vi "Network Steam Create.vi"(8 "error in (no error)":errorcluster, 11 "Model_AMC in":refnum<class "Model_AMC.lvclass">) -> (0 "error out":errorcluster, 3 "Model_AMC out":refnum<class "Model_AMC.lvclass">)   [LabVIEW 2021, in "Model_AMC.lvclass"]
uses:
  Model_AMC.lvclass
  Model_AMC.lvclass/Model_AMC.ctl
  <userlib>/John_Lib/Network_Streams_Connection/NetworkConnection.lvclass
  <userlib>/John_Lib/Network_Streams_Connection/PublicSettings.ctl
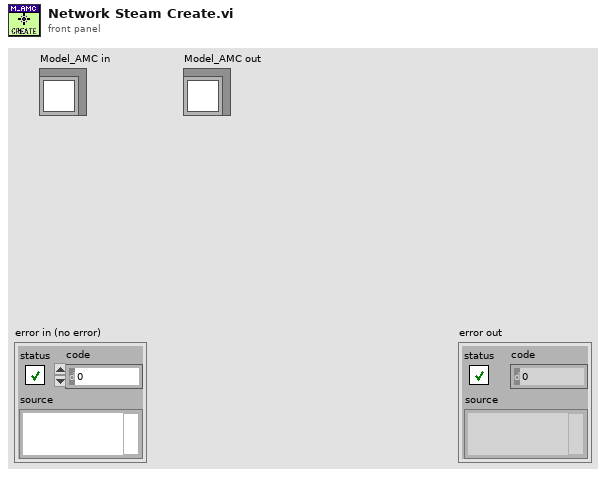
[diagram p1: front panel]
types:
  T1 = typedef "JKI_Network_Streams.lvlib/NetworkConnection.lvclass/PublicSettings.ctl" = cluster{"My Name":string, "Remote IP Address":string, "Remote Name":string}
  T2 = typedef "Model_AMC.lvclass/DVR.ctl" = cluster{"JKI_Network_Streams":refnum<class "NetworkConnection.lvclass">, "AMC Q":T3, "Connnected":bool}
  T3 = typedef "Model_AMC.lvclass/AMC Q.ctl" = cluster{"Main":T4, "OPCUA":T4, "NetworkSteam":T4}
  T4 = typedef "AMC_FW.lvlib/Queue.ctl" = cluster{"Q":T5, "Name":string}
  T5 = typedef "AMC_FW.lvlib/Message Queue.ctl" = refnum<queue>
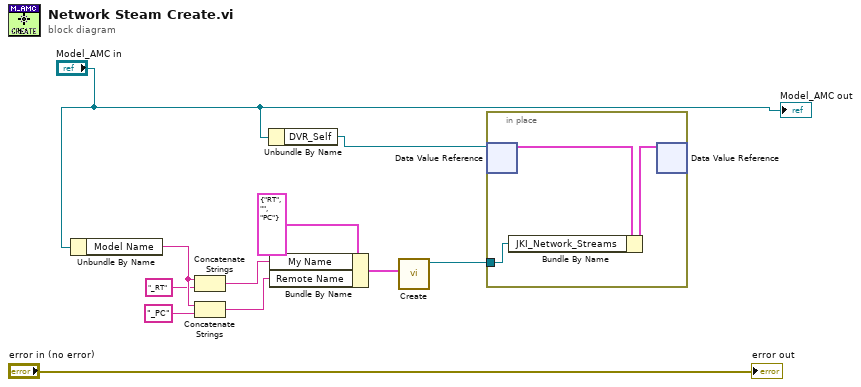
[diagram p0: block diagram]
diagram:
  n1 = Unbundle By Name("Model_AMC in") -> ("Model Name"=w10:string)
  n2 = Concatenate Strings(w10, "_RT" ("string")) -> (w7:string)
  n3 = Concatenate Strings(w10, "_PC" ("string")) -> (w9:string)
  n4 = Unbundle By Name("Model_AMC in") -> ("DVR_Self"=w3:refnum<data-value>)
  n5 = Bundle By Name(cluster=T1 {"My Name"="RT", "Remote IP Address"="", "Remote Name"="PC"} ("Settings"), "My Name"=w7, "Remote Name"=w9) -> (w5:T1)
  n6 = call <userlib>:"Create.vi"("Settings"=w5) -> ("NetworkConnection out"=w2:refnum<class "NetworkConnection.lvclass">)  [unwired: 9 in, 1 out]
  n7 = in-place {
    in-place-border: w2 -> [w12]
    n8 = in-place-dvr #1(w3) -> (w14:T2)  [unwired: 1 out]
    n9 = Bundle By Name(cluster=w14, "JKI_Network_Streams"=w12) -> (w13:T2)
    n10 = in-place-dvr #1(w13) -> ()  [unwired: 2 out]
  }
  "error out" <- "error in (no error)"
  "Model_AMC out" <- "Model_AMC in"
